vi "draw.vi"(8 "error in (no error)":errorcluster, 11 "Rectangle in":refnum<class "Rectangle.lvclass">) -> (0 "error out":errorcluster, 3 "Rectangle out":refnum<class "Rectangle.lvclass">)   [LabVIEW 2018, in "Rectangle.lvclass"]
uses:
  Rectangle.lvclass
  Shape Class/Shape.lvclass
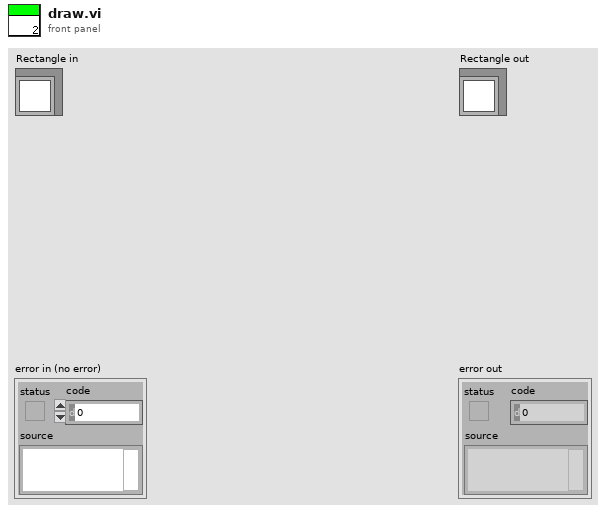
[diagram p1: front panel]
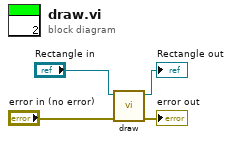
[diagram p0: block diagram]
diagram:
  n1 = call-parent "draw.vi"("error in (no error)"="error in (no error)", "Shape in"="Rectangle in") -> ("error out"=→"error out":errorcluster, "Shape out"=→"Rectangle out":refnum<class "Rectangle.lvclass">)  [unwired: 8 in]
